vi "Write_Wrap_Simple.vi"(4 "Value":T1) -> (1 "Var":refnum<class "Var_U8.lvclass">)   [LabVIEW 2021, in "Var_U8.lvclass"]
uses:
  Var_U8.lvclass
  Type.ctl
  Var_U8.lvclass/Var_U8.ctl
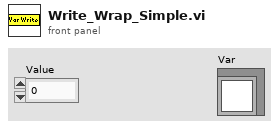
[diagram p1: front panel]
types:
  T1 = typedef "Var_U8.lvclass/Type.ctl" = dbl
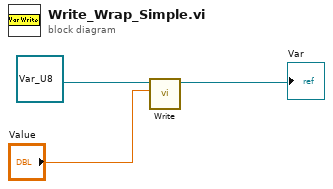
[diagram p0: block diagram]
diagram:
  n1 = call-dynamic "Write.vi"("Value"="Value", "Double Float.lvclass_340760 in"=refnum<class "Var_U8.lvclass"> refnum ("Constants.lvlib:Numeric.lvclass")) -> ("Double Float.lvclass_340760 out"=→"Var":refnum<class "Var_U8.lvclass">)  [unwired: 8 in, 1 out]
